vi "Source Profile Initial Plugin.vi"() -> (5 "Plug in titles":string[](array[string]), 7 "Plug in values":string[](array[string]))   [LabVIEW 2021]
uses:
  Controls/Post_Process.ctl
  Controls/Setup.ctl
  Controls/User_Specific_mode.ctl
  Globals/Trav_pos_global.vi
  Globals/Meas_global.vi
panel:
  out "Profile Filename":path
  in  "Milliseconds between Rendezvous and Acquisition starting":u32
  out "Case Currently On":string
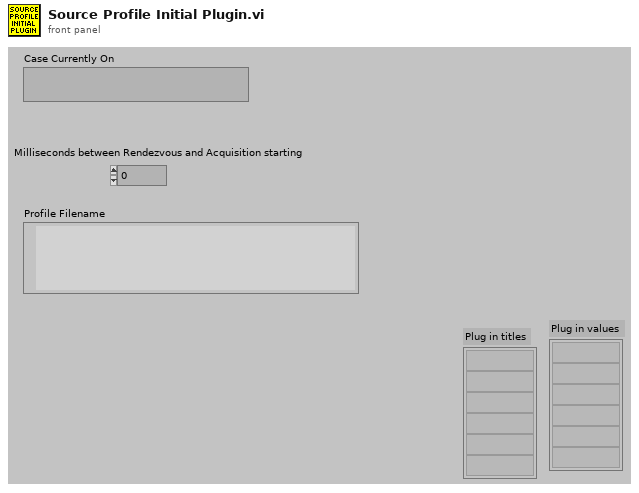
[diagram p1: front panel]
types:
  T1 = typedef "Traverse_cluster.ctl" = cluster{"Start X":sgl, "Start Y":sgl, "Start Z":sgl, "End X":sgl, "End Y":sgl, "End Z":sgl, "nPoints":i32, "Spacing":T2, "Filename":path, "Tunnel Speed":dbl, "Averaging time (mins)":dbl, "Extra Commands":string, "Carrier_1 Q (l/min)":dbl, "Carrier_2 Q (l/min)":dbl, "Trace Gas Concentration (%)":dbl, "Specific Arguments":string, "Comments":string, "Row No":i32, "Row Type Selector":T3, "EstCompl":string, "Row Duration (mins)":dbl, "nValidPoints":i32, "Meas Setup File":string}
  T2 = typedef "Spacing.ctl" = enum16{"Linear", "Log", "Gauss", "Specified", "N/A"}
  T3 = typedef "Multi_run_mode.ctl" = enum16{"Move Traverse Only", "Set Tunnel Speed Only", "Set Source Only", "Set Measurement Conditions", "Single Measurement", "Vertical Profile", "Lateral Profile", "Longitudinal Profile", "Multi-Axis Profile", "Explore Volume", "Auto Calibrate", "Meas Fast FID Bkgnd", "Check Beam Power", "Scanning Valve Measurement", "Run VI Named:", "Set ADAM Ch", "Wait (minutes)", "Send Message", "Synchronize With:", "Fall Back to this Row", "Turn Off Row Repeating", "Traverse 3D Volume", "Blank Row", "Jump to Fall Back Row"}
  T4 = typedef "Setup.ctl" = enum16{"Run Program", "Show Setup", "Save Current Setup", "Setup Front Panel"}
  T5 = typedef "Post_Process.ctl" = enum16{"Take New Data", "Post Process Raw Data File"}
  T6 = typedef "User_Specific_mode.ctl" = enum16{"Check VI only", "Run VI"}
  T7 = typedef "Rendezvous RefNum" = refnum<k1>
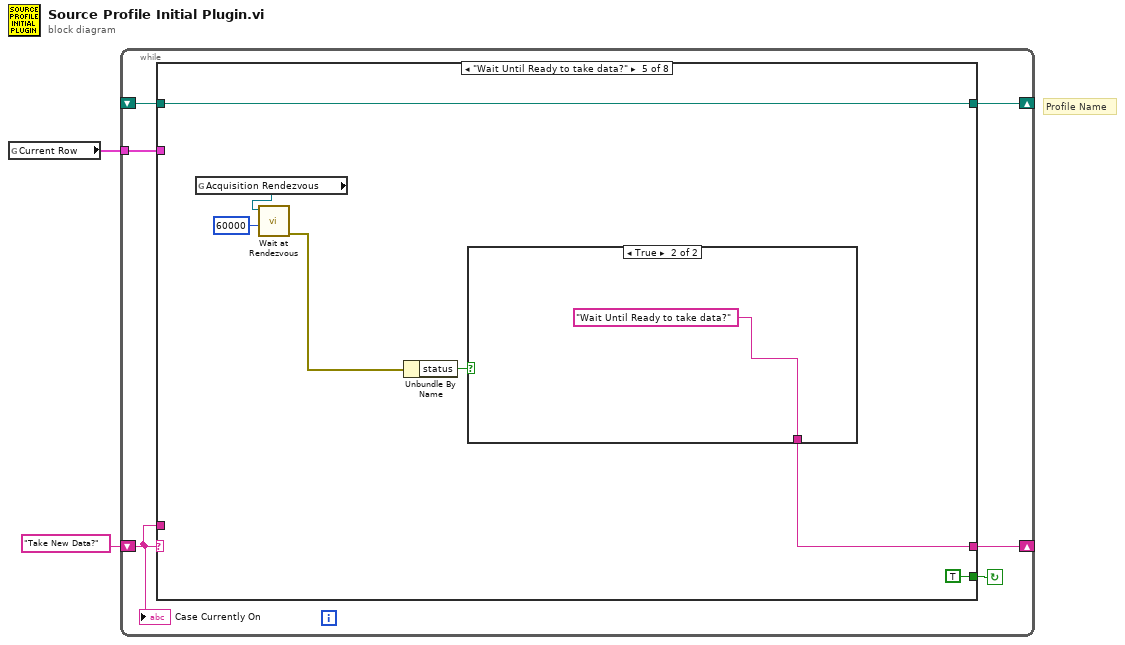
[diagram p0: block diagram]
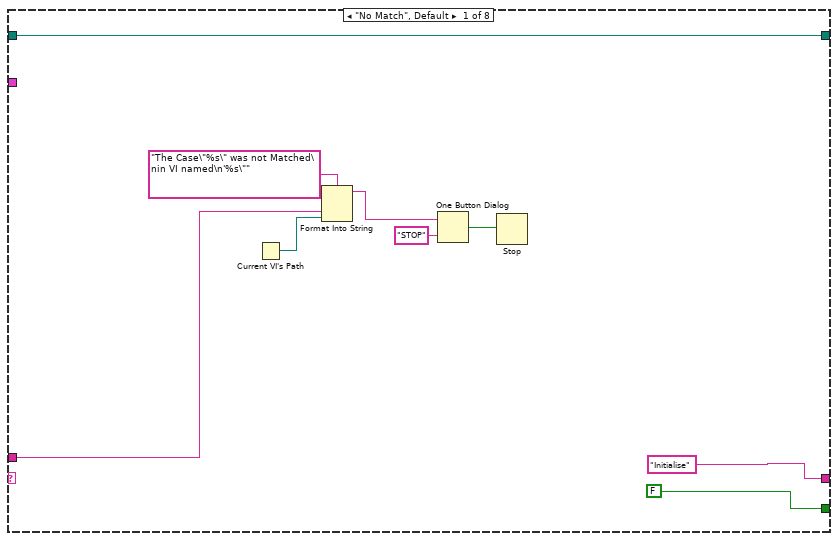
[diagram p2: hidden frame]
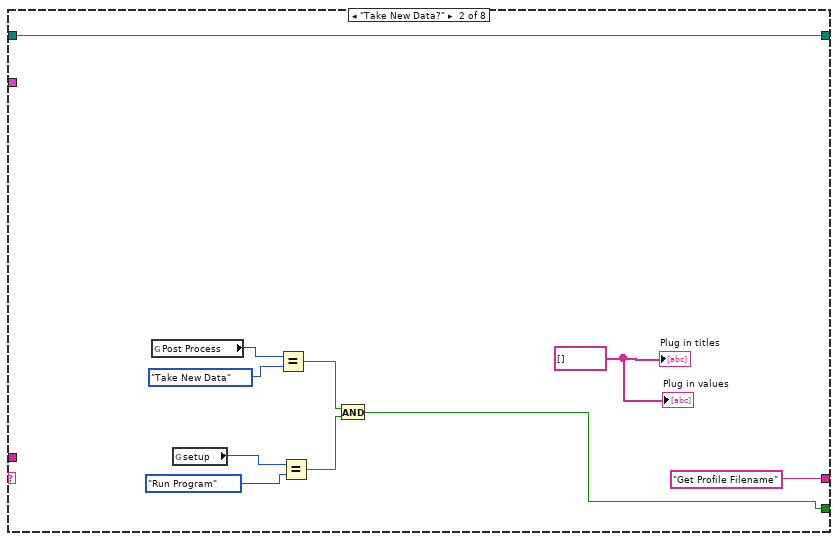
[diagram p3: hidden frame]
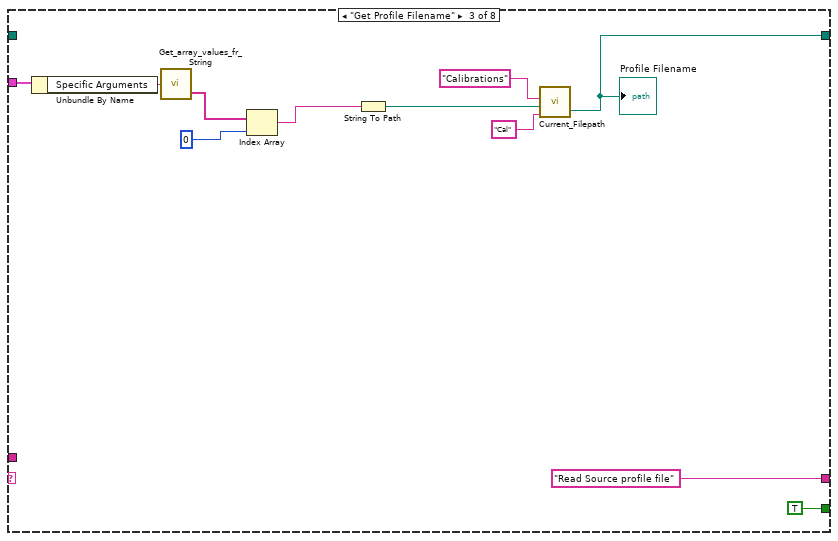
[diagram p4: hidden frame]
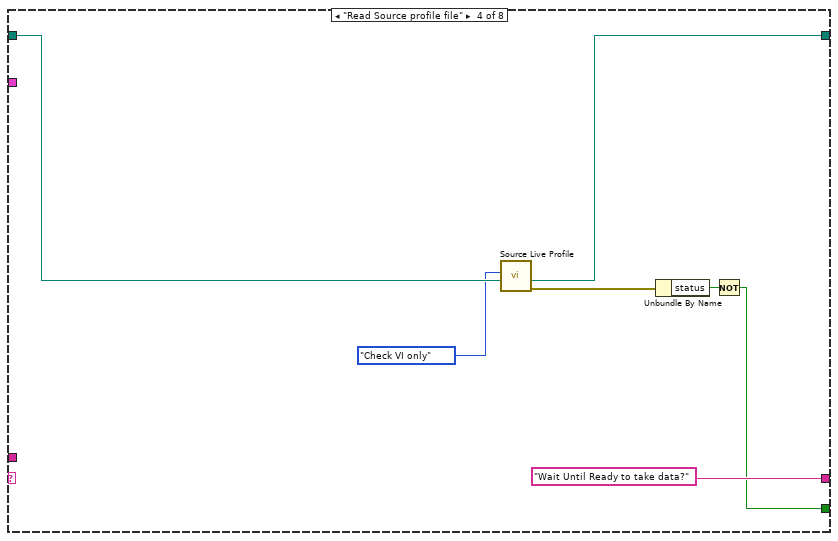
[diagram p5: hidden frame]
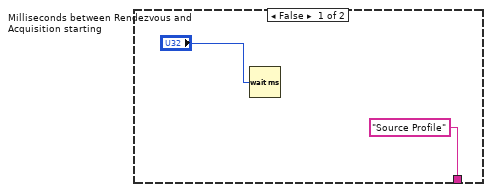
[diagram p6: hidden frame]
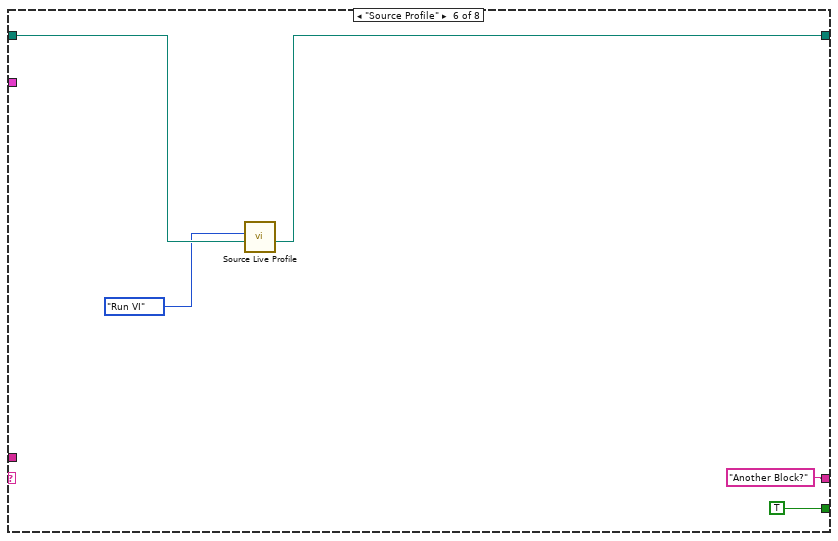
[diagram p7: hidden frame]
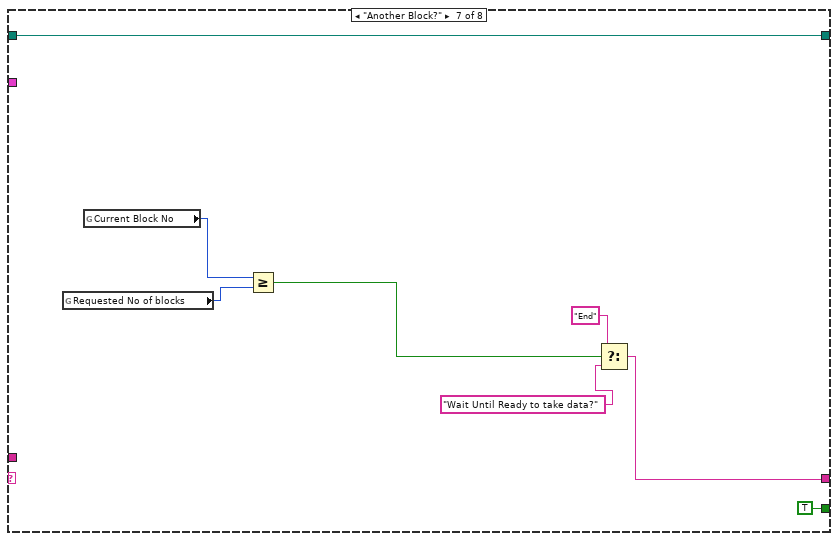
[diagram p8: hidden frame]
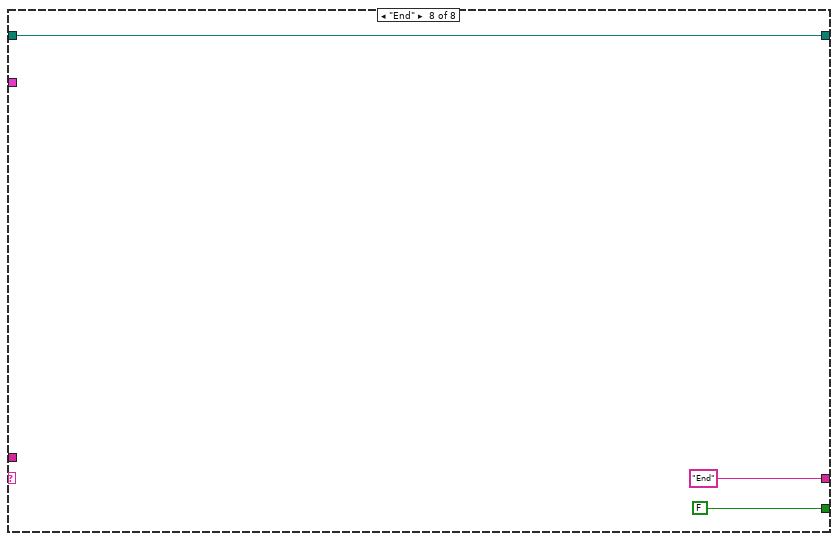
[diagram p9: hidden frame]
diagram:
  # "Profile Name"
  n1 = global read "Trav_pos_global.vi" "Current Row"() -> (w1:T1)
  n2 = while {
    shift-left: "Take New Data?" -> [w6]
    shift-right: [w7] -> _
    tunnel: w1 -> [w5]
    shift-right: [w4] -> _
    shift-left: _ -> [w3]
    stop <- w8 continue-if-true
    n3 = case shown="\"Wait Until Ready to take data?\"" w6 {
      tunnel: [FALSE w19 TRUE ("Command Found") w41 TRUE ("Command Found") TRUE ("Command Found") TRUE ("Command Found") FALSE ("Command Found")] -> w8
      tunnel: ["Initialise" "Get Profile Filename" "Read Source profile file" ("f") "Wait Until Ready to take data?" ("f") w47 "Another Block?" w64 "End" ("f")] -> w7
      tunnel: w6 -> [w12 _ _ _ _ _ _ _]
      tunnel: w5 -> [_ _ w37 _ _ _ _ _]
      tunnel: [w9 w18 w28 w40 w48 w56 w61 w69] -> w4
      tunnel: w3 -> [w9 w18 _ w44 w48 w58 w61 w69]
      frame "No Match", Default {
        n4 = Current VI's Path() -> (path=w11:path)
        n5 = Format Into String(format string="The Case\"%s\" was not Matched\nin VI named\n'%s\"" ("Format String"), w12, w11) -> (resulting string=w15:string)  [unwired: 2 in, 1 out]
        n6 = One Button Dialog(message=w15, button name ("OK")="STOP") -> (true=w13:bool)
        n7 = Stop(stop? (T)=w13) -> ()
      }
      frame "Take New Data?" {
        w24 = string[] [] ("Plug in titles")
        n8 = global read "Meas_global.vi" "Post Process"() -> (w26:T5)
        n9 = global read "Meas_global.vi" "setup"() -> (w23:T4)
        n10 = Equal?(x=w26, y=Post_Process."Take New Data" ("Post Process")) -> (x = y?=w20:bool)
        n11 = Equal?(x=w23, y=Setup."Run Program" ("setup")) -> (x = y?=w21:bool)
        n12 = And(x=w20, y=w21) -> (x .and. y?=w19:bool)
        "Plug in titles" <- w24
        "Plug in values" <- w24
      }
      frame "Get Profile Filename" {
        n13 = Unbundle By Name(w37) -> ("Specific Arguments"=w38:string)
        n14 = call "Get_array_values_fr_String.vi"("String Value"=w38) -> ("String array"=w36:string[])  [unwired: 1 out]
        n15 = Index Array(array=w36, index=0) -> (element=w30:string)
        n16 = String To Path(string=w30) -> (path=w29:path)
        n17 = call "Current_Filepath.vi"("Short_Name"="Cal" ("Data Type"), "Filename in"=w29, "Data Type"="Calibrations") -> ("Filename Out"=w28:path)  [unwired: 1 in, 1 out]
        "Profile Filename" <- w28
      }
      frame "Read Source profile file" {
        n18 = call "Source Live Profile.vi"("Source Profile File"=w44, "Simulate/Run"=User_Specific_mode."Check VI only") -> ("error IO"=w39:errorcluster, "Source Profile Out"=w40:path)  [unwired: 8 in]
        n19 = Unbundle By Name(w39) -> ("status"=w42:bool)
        n20 = Not(x=w42) -> (.not. x?=w41:bool)
      }
      frame "Wait Until Ready to take data?" {
        n21 = global read "Meas_global.vi" "Acquisition Rendezvous"() -> (w51:T7)
        n22 = call <vilib>:"Wait at Rendezvous.vi"("ms timeout (-1)"=60000, "rendezvous"=w51) -> ("error out"=w50:errorcluster)  [unwired: 3 in, 2 out]
        n23 = Unbundle By Name(w50) -> ("status"=w49:bool)
        n24 = case shown="True" w49 {
          tunnel: ["Source Profile" "Wait Until Ready to take data?" ("f")] -> w47
          frame False {
            n25 = Wait (ms)(milliseconds to wait="Milliseconds between Rendezvous and Acquisition starting") -> ()  [unwired: 1 out]
          }
          frame True {
          }
        }
      }
      frame "Source Profile" {
        n26 = call "Source Live Profile.vi"("Source Profile File"=w58, "Simulate/Run"=User_Specific_mode."Run VI") -> ("Source Profile Out"=w56:path)  [unwired: 8 in, 1 out]
      }
      frame "Another Block?" {
        n27 = global read "Meas_global.vi" "Requested No of blocks"() -> (w68:i32)
        n28 = global read "Meas_global.vi" "Current Block No"() -> (w62:i32)
        n29 = Greater Or Equal?(x=w62, y=w68) -> (x >= y?=w66:bool)
        n30 = Select(t="End", s=w66, f="Wait Until Ready to take data?") -> (s? t:f=w64:string)
      }
      frame "End" {
      }
    }
    "Case Currently On" <- w6
  }
